vi "USBRS485-INTERFACE.vi"() -> ()   [LabVIEW 2024]
uses:
  <vilib>/Instr/_visa.llb/VISA Configure Serial Port (Instr).vi
panel:
  in  "Numeric":u8=10 format="%x"
  in  "Boolean":bool
  out "read buffer":string
  out "return count":u32
  in  "VISA resource name":refnum<visa-resource-name>
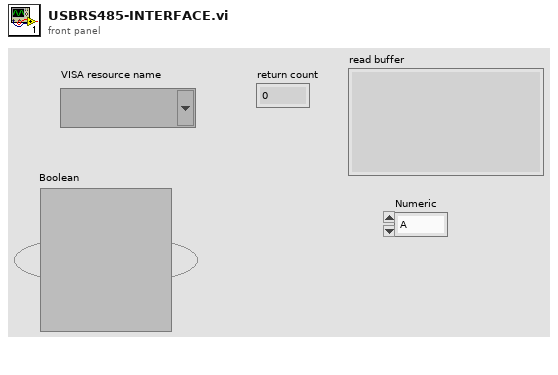
[diagram p1: front panel]
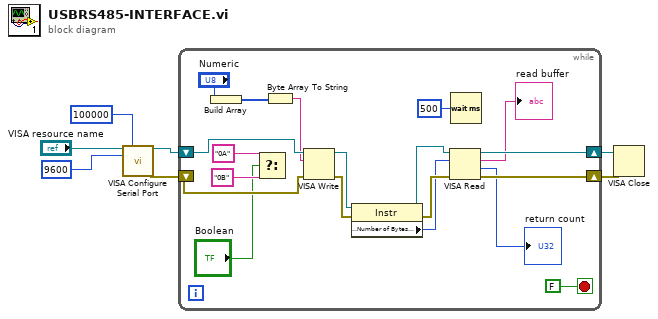
[diagram p0: block diagram]
diagram:
  n1 = call-poly "VISA Configure Serial Port"("VISA resource name"="VISA resource name", "timeout (10sec)"=u32 100000, "baud rate (9600)"=u32 9600) -> ("VISA resource name out"=w5:refnum<visa-resource-name>, "error out"=w2:errorcluster)  [unwired: 11 in]
  n2 = while {
    shift-right: [w23] -> w4
    shift-left: w5 -> [w24]
    shift-right: [w22] -> w3
    shift-left: w2 -> [w21]
    stop <- FALSE stop-if-true
    n3 = Build Array("Numeric") -> (w9:u8[])
    n4 = Select(t="0A", s="Boolean", f="0B") -> ()  [unwired: 1 out]
    n5 = Byte Array To String(unsigned byte array=w9) -> (string=w8:string)
    n6 = VISA Write(VISA resource name=w24, write buffer=w8, error in (no error)=w21) -> (VISA resource name out=w15:refnum<visa-resource-name>, error out=w16:errorcluster)  [unwired: 1 out]
    n7 = property class="Instr"(reference=w15, error in=w16) -> (reference out=w14:refnum<visa-resource-name>, error out=w13:errorcluster, "Serial Settings:Number of Bytes at Serial Port"=w11:u32)
    n8 = VISA Read(VISA resource name=w14, byte count=w11, error in (no error)=w13) -> (VISA resource name out=w23:refnum<visa-resource-name>, read buffer=→"read buffer":string, return count=→"return count":u32, error out=w22:errorcluster)
    n9 = Wait (ms)(milliseconds to wait=u32 500) -> ()  [unwired: 1 out]
  }
  n10 = VISA Close(VISA resource name=w4, error in (no error)=w3) -> ()  [unwired: 1 out]
